vi "Subscribe.vi"(6 "Transport":refnum<class "ITransport.lvclass">, 7 "Unique Subscriber ID":string, 8 "error in (no error)":errorcluster, 9 "Subscription Type":variant, 10 "Subscription Name":string, 11 "ISubject in":refnum<class "ISubject.lvclass">) -> (0 "error out":errorcluster, 3 "ISubject out":refnum<class "ISubject.lvclass">)   [LabVIEW 2015, in "Observer.lvlib" / "ISubject.lvclass"]
uses:
  ISubject.lvclass
  Mediator/Transport/ITransport/ITransport.lvclass
  ISubject.lvclass/ISubject.ctl
  <vilib>/Utility/Data Type/NI_Data Type.lvlib
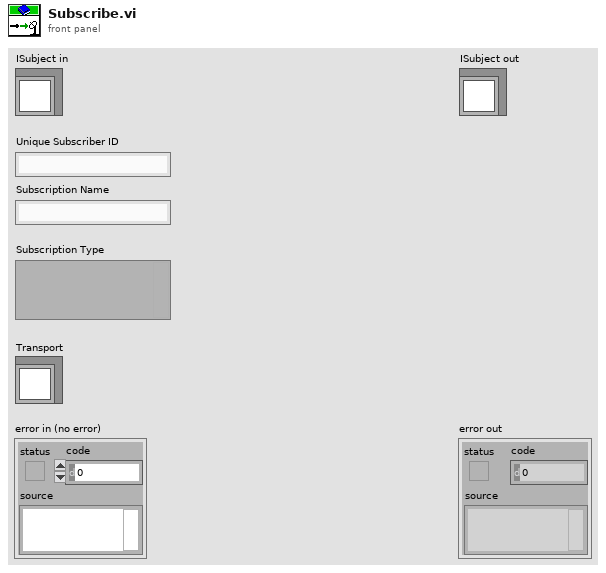
[diagram p1: front panel]
types:
  T1 = typedef "NI_Data Type.lvlib/Data Type.ctl" = enum8{"Invalid Type", "Void", "I8", "I16", "I32", "I64", "U8", "U16", "U32", "U64", "Single Float", "Double Float", "Extended Float", "Single Complex", "Double Complex", "Extended Complex", "Enum U8", "Enum U16", "Enum U32", "Enum U64", "Single Float With Unit", "Double Float With Unit", "Extended Float With Unit", "Single Complex with Unit", "Double Complex with Unit", "Extended Complex with Unit", "Boolean", "String", "Path", "Picture", "Tag", "Array", "Cluster", "Variant", "LV Variant", "Waveform", "Timestamp", "Digital Waveform", "Digital Data", "ExpressData", "Refnum", "External Data", "VI", "Poly VI", "LabVIEW Class Instance", "Fixed Point"}
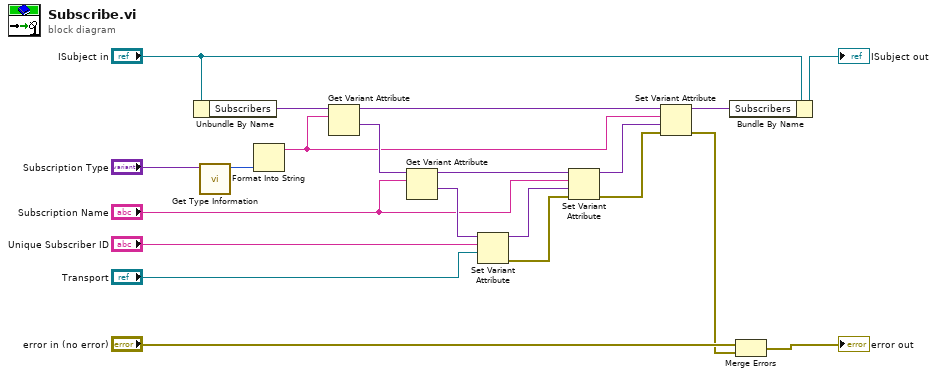
[diagram p0: block diagram]
diagram:
  n1 = Unbundle By Name("ISubject in") -> ("Subscribers"=w18:variant)
  n2 = call <vilib>:"Get Type Information.vi"("Variant"="Subscription Type") -> ("Type"=w17:T1)  [unwired: 6 in, 4 out]
  n3 = Format Into String(w17) -> (resulting string=w13:string)  [unwired: 3 in, 1 out]
  n4 = Get Variant Attribute(Variant=w18, name=w13) -> (duplicate Variant=w16:variant, value=w15:variant)  [unwired: 2 in, 2 out]
  n5 = Get Variant Attribute(Variant=w15, name="Subscription Name") -> (duplicate Variant=w14:variant, value=w11:variant)  [unwired: 2 in, 2 out]
  n6 = Set Variant Attribute(Variant=w11, name="Unique Subscriber ID", value="Transport") -> (Variant out=w10:variant, error out=w6:errorcluster)  [unwired: 1 in, 1 out]
  n7 = Set Variant Attribute(Variant=w14, name="Subscription Name", value=w10, error in=w6) -> (Variant out=w12:variant, error out=w5:errorcluster)  [unwired: 1 out]
  n8 = Set Variant Attribute(Variant=w16, name=w13, value=w12, error in=w5) -> (Variant out=w1:variant, error out=w3:errorcluster)  [unwired: 1 out]
  n9 = Bundle By Name(cluster="ISubject in", "Subscribers"=w1) -> (→"ISubject out":refnum<class "ISubject.lvclass">)
  n10 = Merge Errors("error in (no error)", w3) -> (→"error out":errorcluster)
